vi "Aquire Multi Z-Stack.vi"(4 "#stack":refnum<vi>, 6 "Acquisition Progres Bar":refnum<vi>, 7 "queue in":refnum<queue>, 8 "error in (no error)":errorcluster, 9 "Exp Params":T1={"Experiment Type"="2D Snapshot", "Experiment Name"="Experiment_1", "ExpPath"=path "E:/Data", "TSFrames"=1000, "TSfps"=1000, "ZTSFrames"=1000, "ZTSdt"=1, "Streaming"=FALSE, "Z Stack Settings"={"Start"=0.0, "Step Size"=0.1, "Finish"=1.0}, "total images"=1, "tdms ref"=refnum, "frame #"=0, "images per stack"=1, "total stacks"=1, "period"=1, "PI MVR Increment"=""} {"period" min=1; "total stacks" min=1; "images per stack" min=1; "total images" min=1; "Z Stack Settings"."Start" min=0.0 max=100.0 step=0.1; "Z Stack Settings"."Step Size" min=0.1 max=100.0 step=0.1; "Z Stack Settings"."Finish" min=0.0 max=100.0 step=0.1; "TSFrames" min=1 step=1; "ZTSdt" min=1 step=1; "ZTSFrames" min=2 step=1; "TSfps" min=1 max=1000 step=1}, 10 "PI ID":i32, 11 "pDataBuffer":u16[](array[numeric])) -> (0 "error out":errorcluster, 5 "queue out":refnum<queue>)   [LabVIEW 2020]
uses:
  _Controls/Exp Params.ctl
  _Controls/Logging Queue Cluster.ctl
  _Controls/Tweezertron Ctrl Refs.ctl
  _Controls/Confocal Controls.ctl
  _Controls/iFlex.ctl
  _Controls/PIFOC Position.ctl
  _Controls/Manlight Controls.ctl
  _Controls/Image Thresholds.ctl
  _Controls/Spots.ctl
  <vilib>/Platform/TimedLoop/XDataNode/timing_clust.ctl
  <vilib>/Platform/TimedLoop/XDataNode/nitl_modes.ctl
  <vilib>/Platform/TimedLoop/XDataNode/wakeup.ctl
  _Globals/Global Controls.vi
  <vilib>/Platform/TimedLoop/XDataNode/XDataNode.xnode
  <vilib>/Platform/TimedLoop/XDataNode/XDNodeRunTimeDep.lvlib
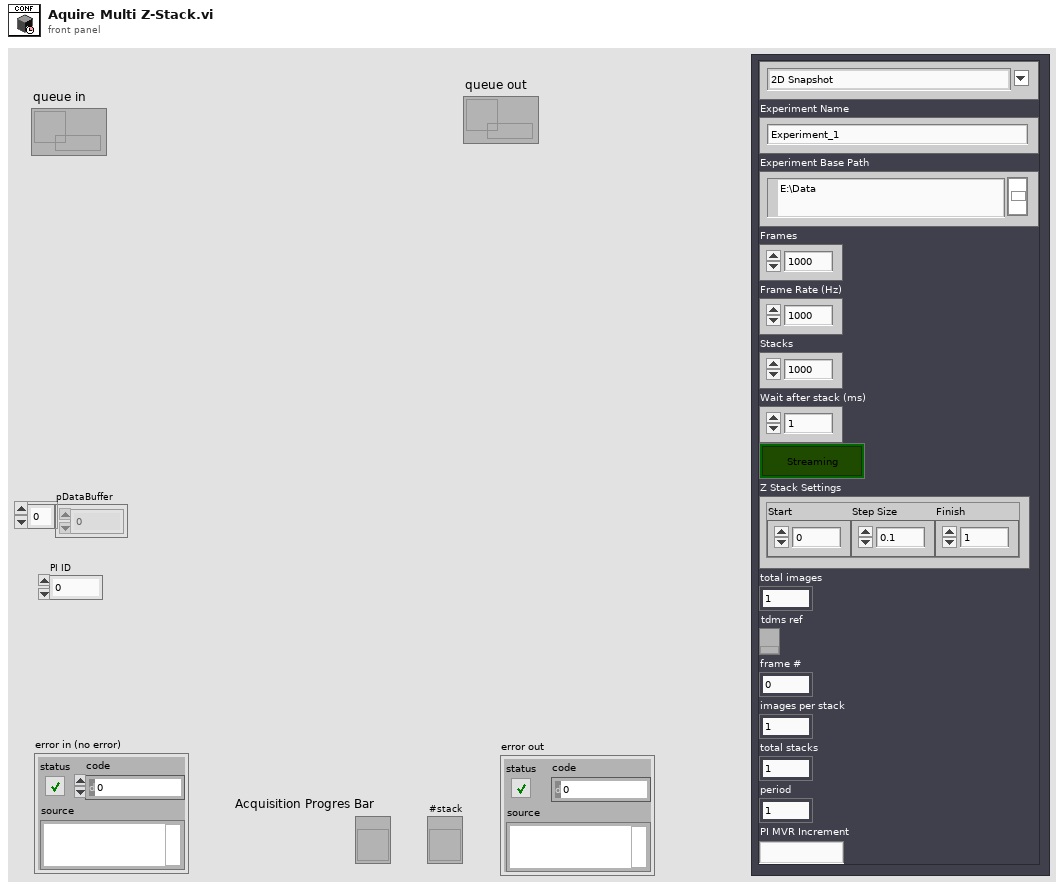
[diagram p1: front panel]
types:
  T1 = typedef "Exp Params.ctl" = cluster{"Experiment Type":string, "Experiment Name":string, "ExpPath":path, "TSFrames":i32, "TSfps":i32, "ZTSFrames":i32, "ZTSdt":i32, "Streaming":bool, "Z Stack Settings":cluster{"Start":dbl, "Step Size":dbl, "Finish":dbl}, "total images":i32, "tdms ref":refnum<k34>, "frame #":i64, "images per stack":i32, "total stacks":i32, "period":i32, "PI MVR Increment":string}
  T2 = typedef "XDNodeRunTimeDep.lvlib/timing_clust.ctl" = cluster{"Expected End [f-1]":u64, "Actual End [f-1]":u64, "Finished Late? [f-1]":bool, "Expected End [i-1]":u64, "Actual End [i-1]":u64, "Finished Late? [i-1]":bool, "Expected Start [i]":u64, "Actual Start [i]":u64, "Expected Start [f]":u64, "Actual Start [f]":u64, "Source Name":string, "Structure Name":string, "Period":i64, "Deadline":i64, "Offset":i64, "Start":i64, "Priority":i32, "Timeout":i32, "Mode":T3, "Wakeup Reason":T4, "Error":errorcluster, "Source Type":string, "Secondary Source Type":string, "Global End Time":u64, "Global Start Time":u64, "Frame Duration":u64, "Iteration Duration":u64, "Assigned CPU":i32, "I/O Scan Engine Mode":u32}
  T3 = typedef "XDNodeRunTimeDep.lvlib/nitl_modes.ctl" = enum32{"No Change", "Process missed periods, maintain original phase", "Discard missed periods, maintain original phase", "Process missed periods, ignore original phase", "Discard missed periods, ignore original phase"}
  T4 = typedef "XDNodeRunTimeDep.lvlib/wakeup.ctl" = enum32{"Normal", "Aborted", "Asynchronous wakeup", "Timing source error", "Timed loop error", "Timeout"}
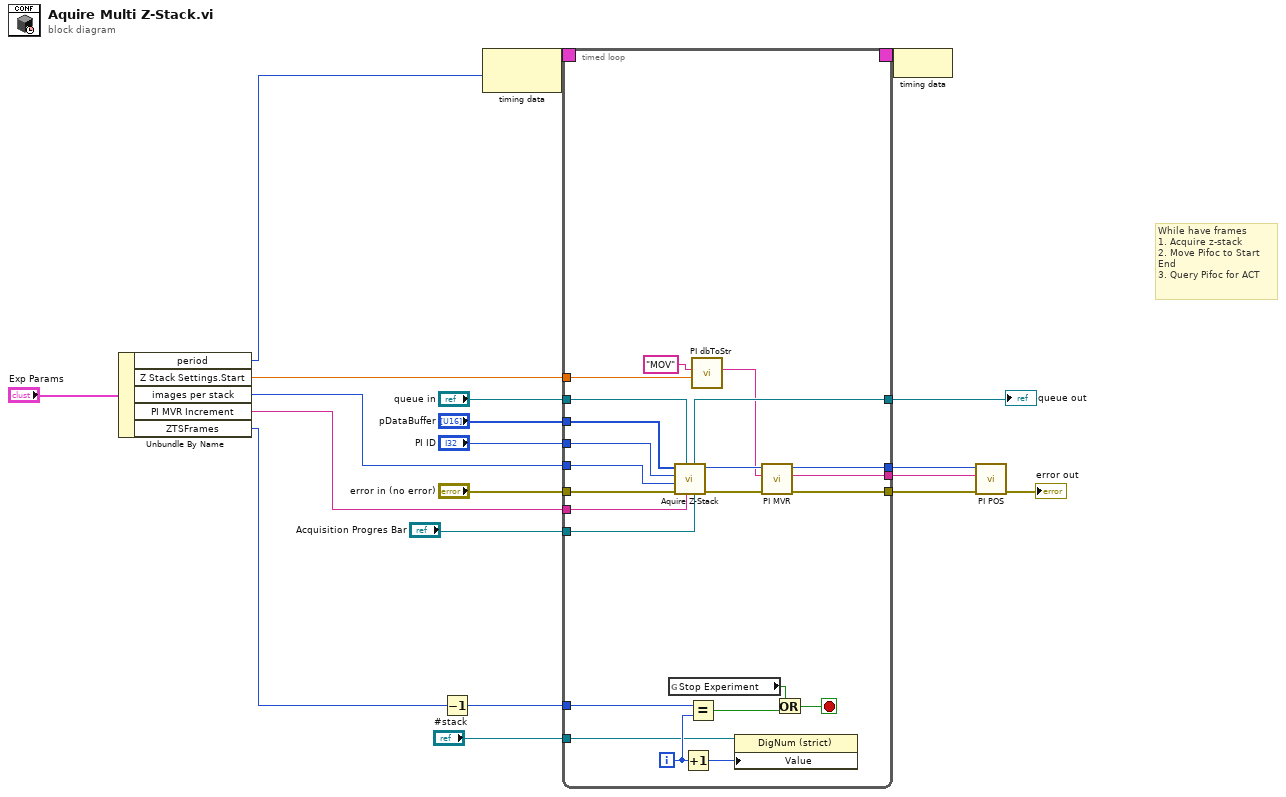
[diagram p0: block diagram]
diagram:
  # "While have frames\n1. Acquire z-stack\n2. Move Pifoc to Start\nEnd\n3. Query Pifoc for ACT"
  n1 = Unbundle By Name("Exp Params") -> ("period"=w5:i32, "Z Stack Settings.Start"=w11:dbl, "images per stack"=w7:i32, "PI MVR Increment"=w6:string, "ZTSFrames"=w4:i32)
  n2 = Decrement(x=w4) -> (x-1=w10:i32)
  n3 = node-c288(w5) -> (w20:T2)
  n4 = timed-loop {
    timing: w20 -> [_]
    timing-out: [_] -> w19
    tunnel: "pDataBuffer" -> [w36]
    tunnel: w6 -> [w33]
    tunnel: w7 -> [w34]
    tunnel: "PI ID" -> [w35]
    tunnel: [w39] -> w16
    tunnel: "error in (no error)" -> [w43]
    tunnel: [w40] -> w17
    tunnel: w10 -> [w42]
    tunnel: w11 -> [w37]
    tunnel: "queue in" -> [w32]
    tunnel: [w30] -> w1
    tunnel: "Acquisition Progres Bar" -> [w31]
    tunnel: "#stack" -> [w28]
    tunnel: [w25] -> w9
    i -> [w29]
    stop <- w22 stop-if-true
    n5 = global read "Global Controls.vi" "Stop Experiment"() -> (w24:bool)
    n6 = call "Aquire Z-Stack.vi"("Acquisition Progres Bar"=w31, "Move Relative Increment"=w33, "queue in"=w32, "error in (no error)"=w43, "Number of slices"=w34, "PI ID in"=w35, "pDataBuffer"=w36) -> ("error out"=w38:errorcluster, "PI ID out"=w27:i32, "queue out"=w30:refnum<queue>)  [unwired: 2 in]
    n7 = Increment(x=w29) -> (x+1=w21:i32)
    n8 = Equal?(x=w42, y=w29) -> (x = y?=w23:bool)
    n9 = call "PI dbToStr.vi"("Start"=w37, "String in"="MOV") -> ("String out"=w26:string)  [unwired: 9 in]
    n10 = property class="DigNum (strict)"(reference=w28, "Value"=w21) -> ()  [unwired: 1 in, 2 out]
    n11 = call "PI MVR.vi"("error in (no error)"=w38, "String"=w26, "PI ID in"=w27) -> ("error out"=w40:errorcluster, "szCommand"=w39:string, "PI ID out"=w25:i32)  [unwired: 6 in]
    n12 = Or(x=w24, y=w23) -> (x .or. y?=w22:bool)
  }
  "queue out" <- w1
  n13 = node-c288(w19) -> ()
  n14 = call "PI POS.vi"("error in (no error)"=w17, "query"=w16, "ID in"=w9) -> ("error out"=→"error out":errorcluster)  [unwired: 6 in, 2 out]
